vi "New.vi"(8 "error in (no error)":errorcluster, 11 "MyData":string) -> (0 "error out":errorcluster, 3 "TipPanelExample out":refnum<class "TipPanelExample.lvclass">)   [LabVIEW 2021, in "TipStripOOPanelExample.lvlib" / "TipPanelExample.lvclass"]
uses:
  TipPanelExample.lvclass
  TipPanelExample.lvclass/TipPanelExample.ctl
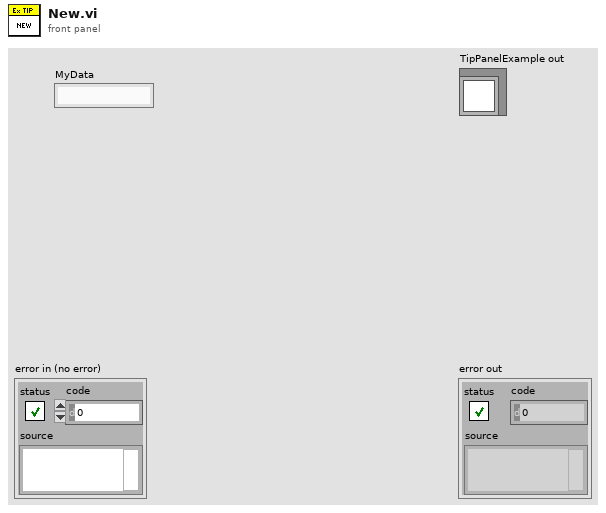
[diagram p1: front panel]
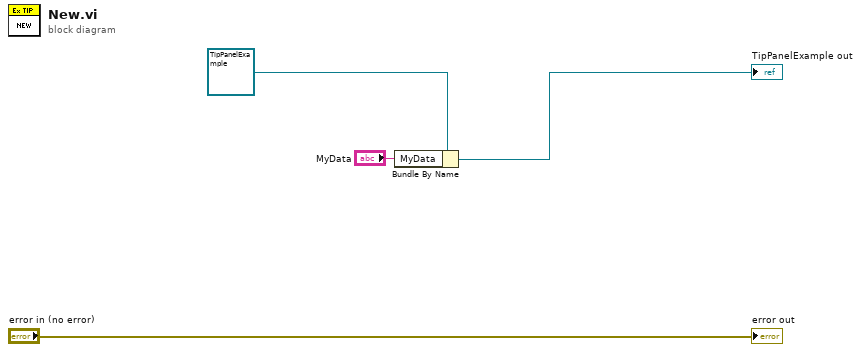
[diagram p0: block diagram]
diagram:
  n1 = Bundle By Name(cluster=refnum<class "TipPanelExample.lvclass"> refnum ("TipPanelExample out"), "MyData"="MyData") -> (→"TipPanelExample out":refnum<class "TipPanelExample.lvclass">)
  "error out" <- "error in (no error)"
